vi "Set theme path.vi"(8 "error in":errorcluster, 10 "theme path":path, 11 "Theme Config in":refnum<class "Theme Config.lvclass">) -> (0 "error out":errorcluster, 3 "Theme Config out":refnum<class "Theme Config.lvclass">)   [LabVIEW 2021, in "Theme Config.lvclass"]
doc: "data member access:\n\nset the theme path\n\n<b>Code Developed By:</b> +\nDaniel Coons +\nTechnology Service Corporation +\nwww.tsc.com/atcs"
uses:
  Theme Config.lvclass
  Theme Config.lvclass/Theme Config.ctl
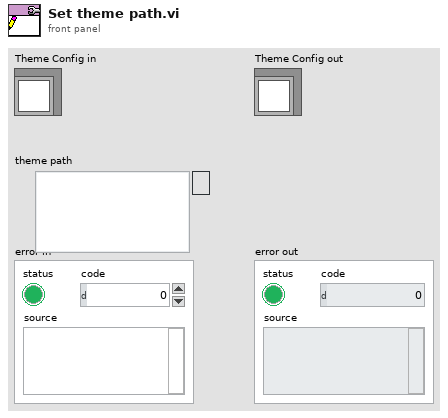
[diagram p1: front panel]
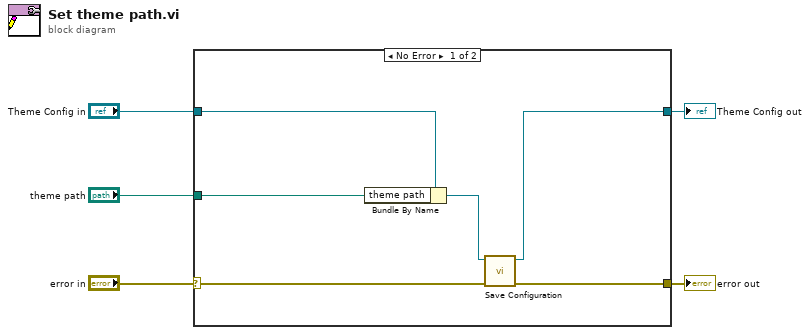
[diagram p0: block diagram]
diagram:
  n1 = case shown="No Error" "error in" {
    selector: "error in" -> [w6 w13]
    tunnel: "Theme Config in" -> [w11 w12]
    tunnel: "theme path" -> [w10 _]
    tunnel: [w9 w13] -> w3
    tunnel: [w7 w12] -> w2
    frame No Error {
      n2 = Bundle By Name(cluster=w11, "theme path"=w10) -> (w8:refnum<class "Theme Config.lvclass">)
      n3 = call "Save Configuration.vi"("error in"=w6, "Theme Config in"=w8) -> ("error out"=w9:errorcluster, "Theme Config out"=w7:refnum<class "Theme Config.lvclass">)  [unwired: 8 in]
    }
    frame Error {
    }
  }
  "error out" <- w3
  "Theme Config out" <- w2
